vi "Set Channel Output.vi"(8 "error in (no error)":errorcluster, 9 "Channel Select":enum16{"Channel 1", "Channel 2", "Channel 3"}(ring), 10 "Enable Output (T: On)":bool=TRUE, 11 "2230G in":refnum<class "2230G.lvclass">) -> (0 "error out":errorcluster, 3 "2230G out":refnum<class "2230G.lvclass">)   [LabVIEW 2018, in "2230G.lvlib" / "2230G.lvclass"]
uses:
  2230G.lvclass
  PPLs/Power Supply/Parent/Power_Supply.lvlibp/Power Supply.lvclass
  <instrlib>/Keithley KE22xx Series/Keithley KE22xx Series.lvlib
  C:/Projects/LabVIEW/PPLs/Power Supply/Parent/Power_Supply.lvlibp/Power Supply.lvclass
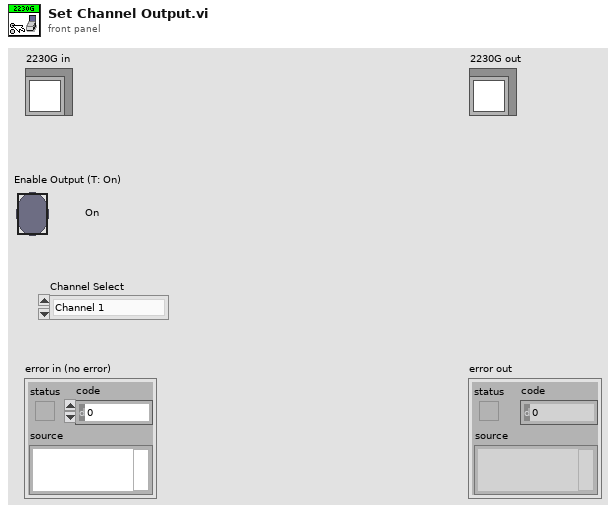
[diagram p1: front panel]
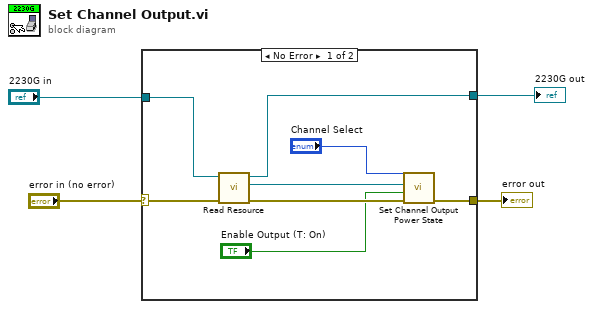
[diagram p0: block diagram]
diagram:
  n1 = case shown="No Error" "error in (no error)" {
    selector: "error in (no error)" -> [w11 w14]
    tunnel: [w8 w14] -> w2
    tunnel: [w10 w13] -> w3
    tunnel: "2230G in" -> [w12 w13]
    frame No Error {
      n2 = call "Read Resource.vi"("error in"=w11, "Power Supply in"=w12) -> ("error out"=w9:errorcluster, "Resource"=w7:refnum<visa-resource-name>, "Power Supply out"=w10:refnum<class "2230G.lvclass">)  [unwired: 7 in]
      n3 = call <instrlib>:"Set Channel Output Power State.vi"("error in (no error)"=w9, "Enable Output (T: On)"="Enable Output (T: On)", "Channel Select"="Channel Select", "Visa Resource Name IN"=w7) -> ("error out"=w8:errorcluster)  [unwired: 6 in, 1 out]
    }
    frame Error {
    }
  }
  "error out" <- w2
  "2230G out" <- w3
